vi "ini Write Key.vi"(0 "Refnum in":T1, 1 "Section":string, 2 "Key":string, 3 "Value":string, 5 "Error In":errorcluster) -> (14 "Refnum Out":T1, 19 "error out":errorcluster)   [LabVIEW 2016, in "Application.lvclass"]
uses:
  Application.lvclass
  <vilib>/Utility/config.llb/Config Data RefNum.ctl
  <vilib>/Utility/config.llb/Write Key (String).vi
  <vilib>/Utility/config.llb/NI_LVConfig.lvlib
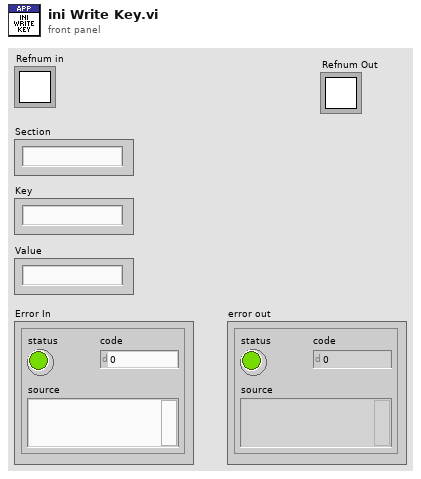
[diagram p1: front panel]
types:
  T1 = typedef "NI_LVConfig.lvlib/Config Data RefNum.ctl" = refnum<k1>
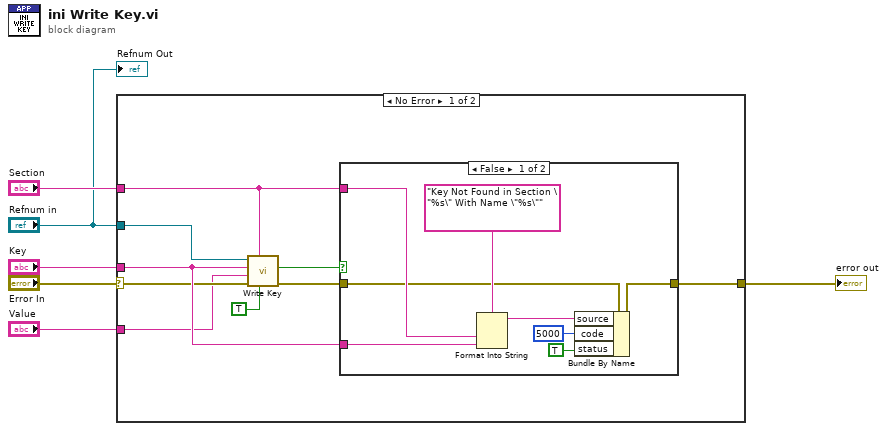
[diagram p0: block diagram]
diagram:
  n1 = case shown="No Error" "Error In" {
    selector: "Error In" -> [w9 w25]
    tunnel: [w15 w25] -> w6
    tunnel: "Refnum in" -> [w12 _]
    tunnel: "Key" -> [w11 _]
    tunnel: "Section" -> [w10 _]
    tunnel: "Value" -> [w8 _]
    frame No Error {
      n2 = call-poly <vilib>:"Write Key.vi"("write raw string? (F)"=TRUE, "section"=w10, "error in (no error)"=w9, "value"=w8, "key"=w11, "refnum"=w12) -> ("error out"=w13:errorcluster, "found?"=w14:bool)  [unwired: 3 in, 1 out]
      n3 = case shown="False" w14 {
        tunnel: w13 -> [w20 w24]
        tunnel: [w18 w24] -> w15
        tunnel: w11 -> [w22 _]
        tunnel: w10 -> [w23 _]
        frame False {
          n4 = Format Into String(format string="Key Not Found in Section \"%s\" With Name \"%s\"", w23, w22) -> (resulting string=w19:string)  [unwired: 2 in, 1 out]
          n5 = Bundle By Name(cluster=w20, "source"=w19, "code"=5000, "status"=TRUE) -> (w18:errorcluster)
        }
        frame True {
        }
      }
    }
    frame Error {
    }
  }
  "error out" <- w6
  "Refnum Out" <- "Refnum in"
